vi "Begin.vi"(8 "error in":errorcluster) -> (0 "error out":errorcluster)   [LabVIEW 2017]
doc: "Called before other user functions, this VI is expected to open initial I/O refnums, load in file data, and do all program initialization. Notice that the <B>error out</B> terminal is simply used for data flow. Wiring it to other structures or subVIs ensures that this VI runs first."
uses:
  <vilib>/Rock Robotics/WPI/SafetyOutput/WPI_SafetyOutputConfigMenu.ctl
  <vilib>/Rock Robotics/WPI/DriverStation/WPI_DriverStationRobotMode2.ctl
  <vilib>/Rock Robotics/WPI/Joystick/WPI_JoystickDeviceEnum.ctl
  <vilib>/Rock Robotics/SystemInterfaces/DIO/FPGA_DIOPWMChannel.ctl
  <vilib>/Rock Robotics/WPI/Solenoid/WPI_SolenoidChannel.ctl
  <vilib>/Rock Robotics/SystemInterfaces/DIO/FPGA_DIOChannel.ctl
  <vilib>/Rock Robotics/WPI/Encoder/WPI_EncoderType.ctl
  Robot Global Data.vi
  <vilib>/Rock Robotics/Network Tables/NT Write String Array.vi
  <vilib>/Rock Robotics/WPI/MotorControl/WPI_MotorControlOpen SPARK.vi
  <vilib>/Rock Robotics/WPI/Utilities/WPI_GetSetVariantRefNum.vi
  <vilib>/Rock Robotics/WPI/Solenoid/WPI_SolenoidOpenSingle.vi
  <vilib>/Rock Robotics/WPI/Counter/WPI_CounterDigitalInputToDigitalSource.vi
  <vilib>/Rock Robotics/WPI/RobotDrive/WPI_RobotDriveOpen4MotorWithSPARK.vi
panel:
  out "Right encoder factor":dbl
  out "Comp. Running":bool
  out "Enabled":bool
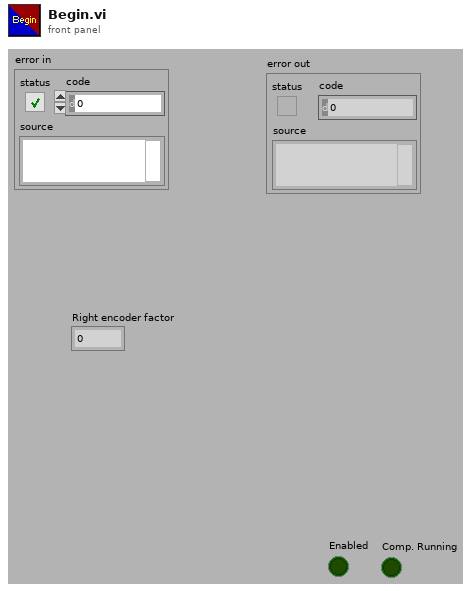
[diagram p1: front panel]
types:
  T1 = typedef "FPGA_DIOPWMChannel.ctl" = enum8{"PWM 0", "PWM 1", "PWM 2", "PWM 3", "PWM 4", "PWM 5", "PWM 6", "PWM 7", "PWM 8", "PWM 9", "PWM MXP 0", "PWM MXP 1", "PWM MXP 2", "PWM MXP 3", "PWM MXP 4", "PWM MXP 5", "PWM MXP 6", "PWM MXP 7", "PWM MXP 8", "PWM MXP 9", "Invalid"}
  T2 = typedef "WPI_EncoderType.ctl" = enum16{"1x", "2x", "4x"}
  T3 = typedef "FPGA_DIOChannel.ctl" = enum8{"DIO 0", "DIO 1", "DIO 2", "DIO 3", "DIO 4", "DIO 5", "DIO 6", "DIO 7", "DIO 8", "DIO 9", "DIO MXP 0", "DIO MXP 1", "DIO MXP 2", "DIO MXP 3", "DIO MXP 4", "DIO MXP 5", "DIO MXP 6", "DIO MXP 7", "DIO MXP 8", "DIO MXP 9", "DIO MXP 10", "DIO MXP 11", "DIO MXP 12", "DIO MXP 13", "DIO MXP 14", "DIO MXP 15", "SPI Port CS1", "SPI Port CS2", "SPI Port CS3", "SPI Port MISO", "SPI Port MOSI", "Invalid"}
  T4 = typedef "WPI_JoystickDeviceEnum.ctl" = enum16{"USB 0", "USB 1", "USB 2", "USB 3", "USB 4", "USB 5"}
  T5 = typedef "WPI_SolenoidChannel.ctl" = enum8{"Solenoid 0", "Solenoid 1", "Solenoid 2", "Solenoid 3", "Solenoid 4", "Solenoid 5", "Solenoid 6", "Solenoid 7", "Invalid"}
  T6 = typedef "WPI_DriverStationRobotMode2.ctl" = enum16{"Autonomous Disabled", "Autonomous Enabled", "Teleop Disabled", "Teleop Enabled", "Disconnected", "Finish", "Test Disabled", "Test Enabled", "Emergency Stopped"}
  T7 = typedef "WPI_SafetyOutputConfigMenu.ctl" = enum16{"Enable", "Disable"}
  T8 = typedef "WPI_RobotDriveDevRef.ctl" = cluster{"DevStatus":errorcluster, "Motors[]":T9[], "Square Inputs":bool, "Max Output":dbl}
  T9 = typedef "WPI_MotorControlDeviceRef.ctl" = cluster{"DeviceStatus":errorcluster, "Type":T10, "PWM":cluster{"PWM Channel":T1, "DeadBand":T11}, "CAN":cluster{"Device Number":u8, "SetOutput VI Ref":variant, "GetOutput VI Ref":variant, "Enable VI Ref":variant, "Disable VI Ref":variant, "Data":variant}, "Invert":bool, "DIO PWM":cluster{"PWM \"Enable\" Channel":T1, "DIOChannel":T3, "PWM Rate":dbl}}
  T10 = typedef "WPI_MotorControlType.ctl" = enum16{"PWM", "CAN", "DIO PWM"}
  T11 = typedef "WPI_PWMDeadband.ctl" = cluster{"Name":string, "maxPositivePwm":i32, "minPositivePwm":i32, "centerPwm":i32, "maxNegativePwm":i32, "minNegativePwm":i32, "angularRange":u16}
  T12 = typedef "WPI_DigitalInputDevRef.ctl" = cluster{"DevStatus":errorcluster, "DIO Channel":T3}
  T13 = typedef "FPGA_CounterEncoderSourceConvertionLVSourceType.ctl" = cluster{"DevStatus":errorcluster, "AnalogTriggerMode?":bool, "DigitalMode":cluster{"DIO Channel":T14}, "AnalogTriggerMode":cluster{"AnalogTriggerIndex":T15, "OutputType":T16}}
  T14 = typedef "FPGA_DIODigitalSourceChannel.ctl" = enum8{"DIO 0", "DIO 1", "DIO 2", "DIO 3", "DIO 4", "DIO 5", "DIO 6", "DIO 7", "DIO 8", "DIO 9", "DIO MXP 0", "DIO MXP 1", "DIO MXP 2", "DIO MXP 3", "DIO MXP 4", "DIO MXP 5", "DIO MXP 6", "DIO MXP 7", "DIO MXP 8", "DIO MXP 9", "DIO MXP 10", "DIO MXP 11", "DIO MXP 12", "DIO MXP 13", "DIO MXP 14", "DIO MXP 15", "Disabled"}
  T15 = typedef "FPGA_AnalogTriggerIndex.ctl" = enum8{"Trig 0", "Trig 1", "Trig 2", "Trig 3", "Trig 4", "Trig 5", "Trig 6", "Trig 7", "Invalid"}
  T16 = typedef "FPGA_AnalogTriggerOutType.ctl" = enum16{"InWindow", "TriggerState", "Rising", "Falling"}
  T17 = typedef "WPI_EncoderDevRef.ctl" = cluster{"DevStatus":errorcluster, "EncoderIndex":T18, "CounterIndex":T19, "DistancePerCount":dbl, "Decoding Type":T2}
  T18 = typedef "FPGA_EncoderIdx.ctl" = enum8{"Enc 0", "Enc 1", "Enc 2", "Enc 3", "Enc 4", "Enc 5", "Enc 6", "Enc 7", "Invalid"}
  T19 = typedef "FPGA_CounterCtrSystemIndex.ctl" = enum8{"Ctr 0", "Ctr 1", "Ctr 2", "Ctr 3", "Ctr 4", "Ctr 5", "Ctr 6", "Ctr 7", "Invalid"}
  T20 = typedef "WPI_CompressorDevRef.ctl" = cluster{"DevStatus":errorcluster, "Pneumatics Control Module":u8}
  T21 = typedef "WPI_SolenoidDevRef.ctl" = cluster{"DevStatus":errorcluster, "Pneumatics Control Module":u8, "Forward Solenoid Channel":T5, "Reverse Solenoid Channel":T5}
  T22 = typedef "WPI_JoystickDevRef.ctl" = cluster{"Device":T4}
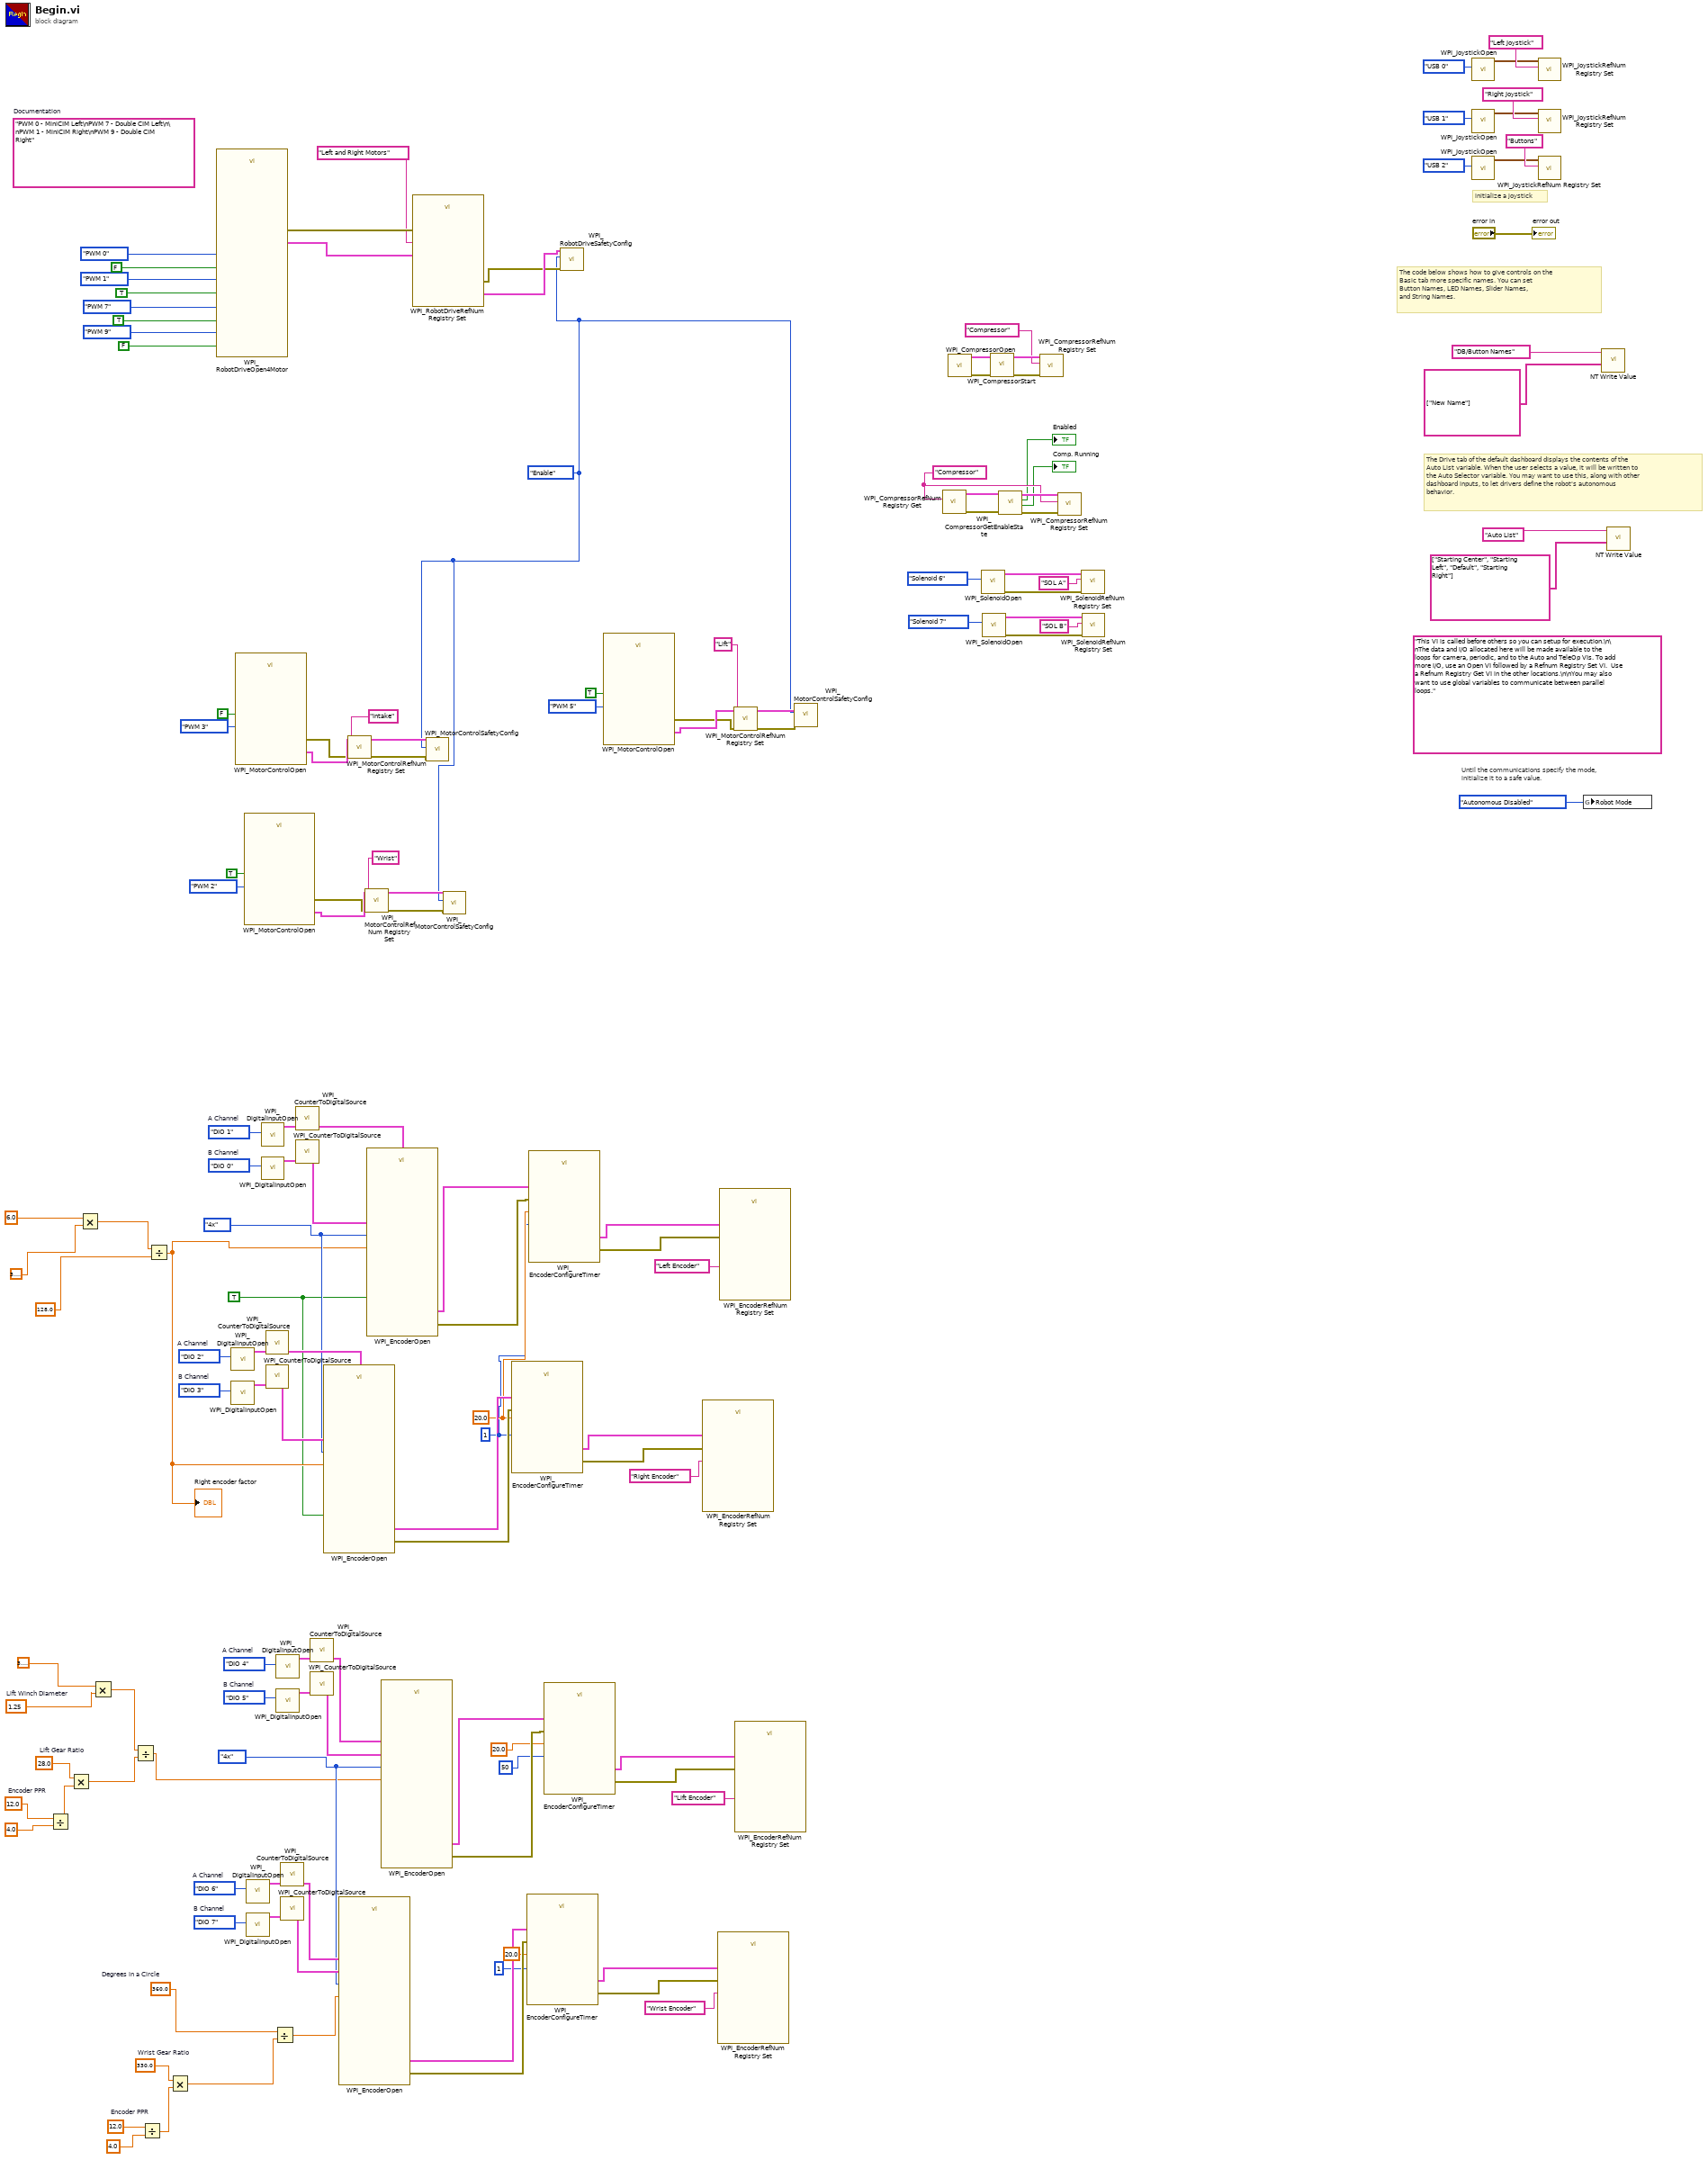
[diagram p0: block diagram]
diagram:
  w1 = TRUE
  w10 = 360.0  # Degrees in a Circle
  w7 = 12.0  # Encoder PPR
  w12 = 330.0  # Wrist Gear Ratio
  (unwired) "PWM 0 - MiniCIM Left\nPWM 7 - Double CIM Left\n\nPWM 1 - MiniCIM Right\nPWM 9 - Double CIM Right"  # Documentation
  w29 = 1.25  # Lift Winch Diameter
  w8 = 12.0  # Encoder PPR
  w30 = 28.0  # Lift Gear Ratio
  w43 = WPI_EncoderType."4x" ("Decoding Type")
  w49 = FPGA_DIOChannel."DIO 7"  # B Channel
  w48 = FPGA_DIOChannel."DIO 6"  # A Channel
  w55 = FPGA_DIOChannel."DIO 5"  # B Channel
  w54 = FPGA_DIOChannel."DIO 4"  # A Channel
  w67 = u8 1 ("Number Samples to Average")
  w68 = 20.0 ("Minimum Rate")
  w85 = WPI_EncoderType."4x" ("Decoding Type")
  w91 = FPGA_DIOChannel."DIO 3"  # B Channel
  w90 = FPGA_DIOChannel."DIO 2"  # A Channel
  w97 = FPGA_DIOChannel."DIO 0"  # B Channel
  w96 = FPGA_DIOChannel."DIO 1"  # A Channel
  w113 = "Compressor"
  w27 = WPI_SafetyOutputConfigMenu."Enable" ("mode")
  (unwired) "This VI is called before others so you can setup for execution.\n\nThe data and I/O allocated here will be made available to the loops for camera, periodic, and to the Auto and TeleOp VIs. To add more I/O, use an Open VI followed by a Refnum Registry Set VI.  Use a Refnum Registry Get VI in the other locations.\n\nYou may also want to use global variables to communicate between parallel loops."
  # "The Drive tab of the default dashboard displays the contents of the\nAuto List variable. When the user selects a value, it will be written to\nthe Auto Selector variable. You may want to use this, along with other\ndashboard inputs, to let drivers define the robot's autonomous\nbehavior."
  # "The code below shows how to give controls on the\nBasic tab more specific names. You can set\nButton Names, LED Names, Slider Names,\nand String Names."
  # "initialize a joystick"
  # "Until the communications specify the mode,\ninitialize it to a safe value."
  n1 = Divide(x=w8, y=4.0) -> (x/y=w5:dbl)
  n2 = Multiply(x=w30, y=w5) -> (x*y=w17:dbl)
  n3 = Multiply(x=6.0, y=3.141592653589793) -> (x*y=w18:dbl)
  n4 = Multiply(x=3.141592653589793, y=w29) -> (x*y=w16:dbl)
  n5 = Divide(x=w16, y=w17) -> (x/y=w28:dbl)
  n6 = Divide(x=w7, y=4.0) -> (x/y=w6:dbl)
  n7 = Divide(x=w18, y=128.0) -> (x/y=w15:dbl)
  "Right encoder factor" <- w15
  n8 = Multiply(x=w12, y=w6) -> (x*y=w11:dbl)
  n9 = call-poly <vilib>:"WPI_RobotDriveOpen4Motor.vi"("Rear Left Motor"=FPGA_DIOPWMChannel."PWM 7" ("Left Motor"), "Rear Left Motor Inverted"=TRUE ("Left Motor Inverted"), "Rear Right Motor Inverted"=FALSE ("Right Motor Inverted"), "Rear Right Motor"=FPGA_DIOPWMChannel."PWM 9" ("Right Motor"), "Front Left Motor"=FPGA_DIOPWMChannel."PWM 0" ("Left Motor"), "Front Right Motor"=FPGA_DIOPWMChannel."PWM 1" ("Right Motor"), "Front Left Motor Inverted"=FALSE ("Left Motor Inverted"), "Front Right Motor Inverted"=TRUE ("Right Motor Inverted")) -> ("RobotDriveDevRef"=w74:T8, "error out"=w73:errorcluster)  [unwired: 6 in]
  n10 = call <vilib>:"WPI_DigitalInputOpen.vi"("DIO Channel"=w90) -> ("DigitalInputDevRef"=w87:T12)  [unwired: 1 in, 9 out]
  n11 = call <vilib>:"WPI_DigitalInputOpen.vi"("DIO Channel"=w91) -> ("DigitalInputDevRef"=w88:T12)  [unwired: 1 in, 9 out]
  n12 = call-poly <vilib>:"WPI_MotorControlOpen.vi"("Invert"=FALSE, "PWM Channel"=FPGA_DIOPWMChannel."PWM 3") -> ("error out"=w120:errorcluster, "MotorControlDeviceRef"=w122:T9)  [unwired: 8 in]
  n13 = call-poly <vilib>:"WPI_MotorControlOpen.vi"("Invert"=TRUE, "PWM Channel"=FPGA_DIOPWMChannel."PWM 2") -> ("error out"=w119:errorcluster, "MotorControlDeviceRef"=w123:T9)  [unwired: 8 in]
  n14 = call <vilib>:"WPI_DigitalInputOpen.vi"("DIO Channel"=w48) -> ("DigitalInputDevRef"=w45:T12)  [unwired: 1 in, 9 out]
  n15 = call <vilib>:"WPI_DigitalInputOpen.vi"("DIO Channel"=w49) -> ("DigitalInputDevRef"=w46:T12)  [unwired: 1 in, 9 out]
  n16 = call <vilib>:"WPI_DigitalInputOpen.vi"("DIO Channel"=w96) -> ("DigitalInputDevRef"=w93:T12)  [unwired: 1 in, 9 out]
  n17 = call <vilib>:"WPI_DigitalInputOpen.vi"("DIO Channel"=w97) -> ("DigitalInputDevRef"=w94:T12)  [unwired: 1 in, 9 out]
  n18 = call-poly <vilib>:"WPI_CounterToDigitalSource.vi"("DigitalInputDevRef"=w87) -> ("Digital Source"=w86:T13)  [unwired: 6 out]
  n19 = call-poly <vilib>:"WPI_CounterToDigitalSource.vi"("DigitalInputDevRef"=w88) -> ("Digital Source"=w89:T13)  [unwired: 6 out]
  n20 = Divide(x=w10, y=w11) -> (x/y=w9:dbl)
  n21 = call <vilib>:"WPI_DigitalInputOpen.vi"("DIO Channel"=w54) -> ("DigitalInputDevRef"=w51:T12)  [unwired: 1 in, 9 out]
  n22 = call <vilib>:"WPI_DigitalInputOpen.vi"("DIO Channel"=w55) -> ("DigitalInputDevRef"=w52:T12)  [unwired: 1 in, 9 out]
  n23 = call-poly <vilib>:"WPI_CounterToDigitalSource.vi"("DigitalInputDevRef"=w45) -> ("Digital Source"=w44:T13)  [unwired: 6 out]
  n24 = call-poly <vilib>:"WPI_CounterToDigitalSource.vi"("DigitalInputDevRef"=w46) -> ("Digital Source"=w47:T13)  [unwired: 6 out]
  n25 = call-poly <vilib>:"WPI_CounterToDigitalSource.vi"("DigitalInputDevRef"=w93) -> ("Digital Source"=w92:T13)  [unwired: 6 out]
  n26 = call-poly <vilib>:"WPI_CounterToDigitalSource.vi"("DigitalInputDevRef"=w94) -> ("Digital Source"=w95:T13)  [unwired: 6 out]
  n27 = call-poly <vilib>:"WPI_CounterToDigitalSource.vi"("DigitalInputDevRef"=w51) -> ("Digital Source"=w50:T13)  [unwired: 6 out]
  n28 = call-poly <vilib>:"WPI_CounterToDigitalSource.vi"("DigitalInputDevRef"=w52) -> ("Digital Source"=w53:T13)  [unwired: 6 out]
  n29 = call <vilib>:"WPI_EncoderOpen.vi"("DistancePerCount"=w15, "Decoding Type"=w85, "Invert Direction (False)"=w1, "BSource"=w89, "ASource"=w86) -> ("error out"=w79:errorcluster, "EncoderDevRef"=w80:T17)  [unwired: 3 in, 2 out]
  n30 = call <vilib>:"WPI_EncoderOpen.vi"("DistancePerCount"=w9, "Decoding Type"=w43, "BSource"=w47, "ASource"=w44) -> ("error out"=w37:errorcluster, "EncoderDevRef"=w38:T17)  [unwired: 4 in, 2 out]
  n31 = call <vilib>:"WPI_MotorControlRefNum Registry Set.vi"("error in (no error)"=w120, "refnum name"="Intake", "MotorControlDevRef"=w122) -> ("error out"=w128:errorcluster, "MotorControlDevRef"=w129:T9)  [unwired: 7 in]
  n32 = call <vilib>:"WPI_MotorControlRefNum Registry Set.vi"("error in (no error)"=w119, "refnum name"="Wrist", "MotorControlDevRef"=w123) -> ("error out"=w126:errorcluster, "MotorControlDevRef"=w127:T9)  [unwired: 7 in]
  n33 = call <vilib>:"WPI_EncoderOpen.vi"("DistancePerCount"=w15, "Decoding Type"=w85, "Invert Direction (False)"=w1, "BSource"=w95, "ASource"=w92) -> ("error out"=w83:errorcluster, "EncoderDevRef"=w84:T17)  [unwired: 3 in, 2 out]
  n34 = call <vilib>:"WPI_EncoderOpen.vi"("DistancePerCount"=w28, "Decoding Type"=w43, "BSource"=w53, "ASource"=w50) -> ("error out"=w41:errorcluster, "EncoderDevRef"=w42:T17)  [unwired: 4 in, 2 out]
  n35 = call <vilib>:"WPI_RobotDriveRefNum Registry Set.vi"("error in (no error)"=w73, "refnum name"="Left and Right Motors", "RobotDriveDevRef"=w74) -> ("error out"=w69:errorcluster, "RobotDriveDevRef"=w70:T8)  [unwired: 1 in, 6 out]
  n36 = call <vilib>:"WPI_MotorControlSafetyConfig.vi"("error in (no error)"=w128, "mode"=w27, "MotorControlDevRef"=w129) -> ()  [unwired: 7 in, 2 out]
  n37 = call <vilib>:"WPI_MotorControlSafetyConfig.vi"("error in (no error)"=w126, "mode"=w27, "MotorControlDevRef"=w127) -> ()  [unwired: 7 in, 2 out]
  n38 = call <vilib>:"WPI_EncoderConfigureTimer.vi"("error in (no error)"=w79, "Number Samples to Average"=w67, "Minimum Rate"=w68, "EncoderDevRef"=w80) -> ("error out"=w81:errorcluster, "EncoderDevRef"=w82:T17)  [unwired: 6 in]
  n39 = call <vilib>:"WPI_EncoderConfigureTimer.vi"("error in (no error)"=w37, "Number Samples to Average"=1, "Minimum Rate"=20.0, "EncoderDevRef"=w38) -> ("error out"=w39:errorcluster, "EncoderDevRef"=w40:T17)  [unwired: 6 in]
  n40 = call <vilib>:"WPI_EncoderConfigureTimer.vi"("error in (no error)"=w83, "Number Samples to Average"=w67, "Minimum Rate"=w68, "EncoderDevRef"=w84) -> ("error out"=w77:errorcluster, "EncoderDevRef"=w78:T17)  [unwired: 6 in]
  n41 = call <vilib>:"WPI_EncoderConfigureTimer.vi"("error in (no error)"=w41, "Number Samples to Average"=u8 50, "Minimum Rate"=20.0, "EncoderDevRef"=w42) -> ("error out"=w35:errorcluster, "EncoderDevRef"=w36:T17)  [unwired: 6 in]
  n42 = call <vilib>:"WPI_RobotDriveSafetyConfig.vi"("error in (no error)"=w69, "mode"=w27, "RobotDriveDevRef"=w70) -> ()  [unwired: 7 in, 2 out]
  n43 = call-poly <vilib>:"WPI_MotorControlOpen.vi"("Invert"=TRUE, "PWM Channel"=FPGA_DIOPWMChannel."PWM 5") -> ("error out"=w118:errorcluster, "MotorControlDeviceRef"=w121:T9)  [unwired: 8 in]
  n44 = call <vilib>:"WPI_EncoderRefNum Registry Set.vi"("error in (no error)"=w81, "refnum name"="Right Encoder", "EncoderDevRef"=w82) -> ()  [unwired: 7 in, 2 out]
  n45 = call <vilib>:"WPI_EncoderRefNum Registry Set.vi"("error in (no error)"=w39, "refnum name"="Wrist Encoder", "EncoderDevRef"=w40) -> ()  [unwired: 7 in, 2 out]
  n46 = call <vilib>:"WPI_EncoderRefNum Registry Set.vi"("error in (no error)"=w77, "refnum name"="Left Encoder", "EncoderDevRef"=w78) -> ()  [unwired: 7 in, 2 out]
  n47 = call <vilib>:"WPI_MotorControlRefNum Registry Set.vi"("error in (no error)"=w118, "refnum name"="Lift", "MotorControlDevRef"=w121) -> ("error out"=w124:errorcluster, "MotorControlDevRef"=w125:T9)  [unwired: 7 in]
  n48 = call <vilib>:"WPI_EncoderRefNum Registry Set.vi"("error in (no error)"=w35, "refnum name"="Lift Encoder", "EncoderDevRef"=w36) -> ()  [unwired: 7 in, 2 out]
  n49 = call <vilib>:"WPI_MotorControlSafetyConfig.vi"("error in (no error)"=w124, "mode"=w27, "MotorControlDevRef"=w125) -> ()  [unwired: 7 in, 2 out]
  n50 = call <vilib>:"WPI_CompressorRefNum Registry Get.vi"("refnum name"=w113) -> ("error out"=w115:errorcluster, "CompressorDevRef"=w117:T20)  [unwired: 9 in]
  n51 = call <vilib>:"WPI_CompressorOpen.vi"() -> ("CompressorDevRef"=w101:T20, "error out"=w102:errorcluster)  [unwired: 14 in]
  n52 = call-poly <vilib>:"WPI_SolenoidOpen.vi"("Solenoid Channel"=WPI_SolenoidChannel."Solenoid 6") -> ("error out"=w108:errorcluster, "SolenoidDevRef"=w109:T21)  [unwired: 9 in]
  n53 = call-poly <vilib>:"WPI_SolenoidOpen.vi"("Solenoid Channel"=WPI_SolenoidChannel."Solenoid 7") -> ("error out"=w104:errorcluster, "SolenoidDevRef"=w105:T21)  [unwired: 9 in]
  n54 = call <vilib>:"WPI_CompressorStart.vi"("error in (no error)"=w102, "CompressorDevRef"=w101) -> ("error out"=w99:errorcluster, "CompressorDevRef"=w100:T20)  [unwired: 8 in]
  n55 = call <vilib>:"WPI_CompressorGetEnableState.vi"("error in (no error)"=w115, "CompressorDevRef"=w117) -> ("error out"=w114:errorcluster, "Compressor Running"=→"Comp. Running":bool, "Enabled"=→"Enabled":bool, "CompressorDevRef"=w116:T20)  [unwired: 6 in]
  n56 = call <vilib>:"WPI_CompressorRefNum Registry Set.vi"("error in (no error)"=w99, "refnum name"="Compressor", "CompressorDevRef"=w100) -> ()  [unwired: 7 in, 2 out]
  n57 = call <vilib>:"WPI_CompressorRefNum Registry Set.vi"("error in (no error)"=w114, "refnum name"=w113, "CompressorDevRef"=w116) -> ()  [unwired: 7 in, 2 out]
  n58 = call <vilib>:"WPI_SolenoidRefNum Registry Set.vi"("error in (no error)"=w108, "refnum name"="SOL A", "SolenoidDevRef"=w109) -> ()  [unwired: 7 in, 2 out]
  n59 = call <vilib>:"WPI_SolenoidRefNum Registry Set.vi"("error in (no error)"=w104, "refnum name"="SOL B", "SolenoidDevRef"=w105) -> ()  [unwired: 7 in, 2 out]
  n60 = call <vilib>:"WPI_JoystickOpen.vi"("JoystickDevice"=WPI_JoystickDeviceEnum."USB 0") -> ("JoystickDevRef"=w142:T22)  [unwired: 10 in]
  n61 = call <vilib>:"WPI_JoystickOpen.vi"("JoystickDevice"=WPI_JoystickDeviceEnum."USB 1") -> ("JoystickDevRef"=w60:T22)  [unwired: 10 in]
  n62 = call <vilib>:"WPI_JoystickOpen.vi"("JoystickDevice"=WPI_JoystickDeviceEnum."USB 2") -> ("JoystickDevRef"=w57:T22)  [unwired: 10 in]
  n63 = call <vilib>:"WPI_JoystickRefNum Registry Set.vi"("refnum name"="Left Joystick", "JoystickDevRef"=w142) -> ()  [unwired: 8 in, 2 out]
  n64 = call <vilib>:"WPI_JoystickRefNum Registry Set.vi"("refnum name"="Right Joystick", "JoystickDevRef"=w60) -> ()  [unwired: 8 in, 2 out]
  n65 = call <vilib>:"WPI_JoystickRefNum Registry Set.vi"("refnum name"="Buttons", "JoystickDevRef"=w57) -> ()  [unwired: 8 in, 2 out]
  n66 = global write "Robot Global Data.vi" "Robot Mode"(WPI_DriverStationRobotMode2."Autonomous Disabled" ("Robot Mode")) -> ()
  n67 = call-poly <vilib>:"NT Write Value.vi"("String Array"=string[] ["New Name"], "Name"="DB/Button Names") -> ()  [unwired: 9 in, 1 out]
  n68 = call-poly <vilib>:"NT Write Value.vi"("String Array"=string[] ["Starting Center", "Starting Left", "Default", "Starting Right"], "Name"="Auto List") -> ()  [unwired: 9 in, 1 out]
  "error out" <- "error in"
